vi "DashboardTest.vi"() -> ()   [LabVIEW 2020]
uses:
  <vilib>/Rock Robotics/Network Tables/NT Read Number.vi
  <vilib>/Rock Robotics/Network Tables/NT Read String.vi
  <vilib>/Rock Robotics/Network Tables/NT Read Boolean.vi
  <vilib>/vision/NI_Vision_Development_Module.lvlib
panel:
  out "Image 2":T1(plugin-control)
  out "Image":T1(plugin-control)
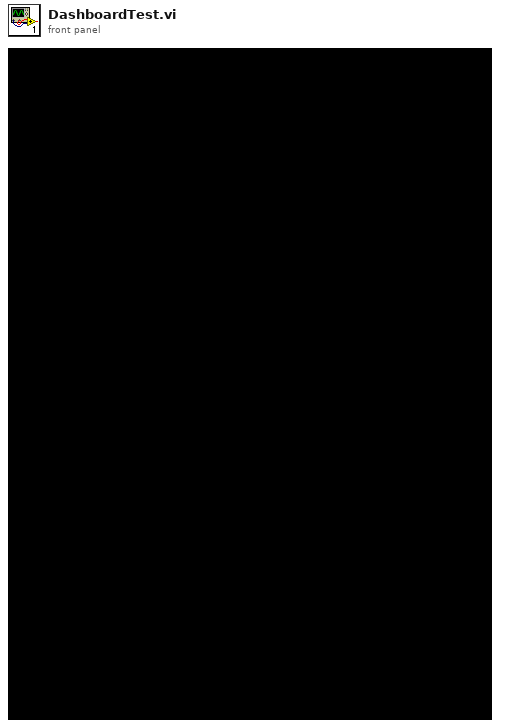
[diagram p1: front panel]
types:
  T1 = typedef "IMAQ Image.ctl" = refnum<image>
  T2 = typedef "Image Type" = u32
  T3 = typedef "LVRectTypeDef.ctl" = cluster{"Left":i16, "Top":i16, "Right":i16, "Bottom":i16}
  T4 = typedef "LVAllMonitorsDisplayTypeDef.ctl" = cluster{"Bounds":cluster{"Left":i16, "Top":i16, "Right":i16, "Bottom":i16}, "Depth":i16}[]
  T5 = cluster{"Left":i16, "Top":i16, "Right":i16, "Bottom":i16}
  T6 = cluster{"Bounds[0]":i16, "Bounds[1]":i16, "Bounds[2]":i16, "Bounds[3]":i16}
  T7 = cluster{"Left":i32, "Top":i32, "Right":i32, "Bottom":i32}
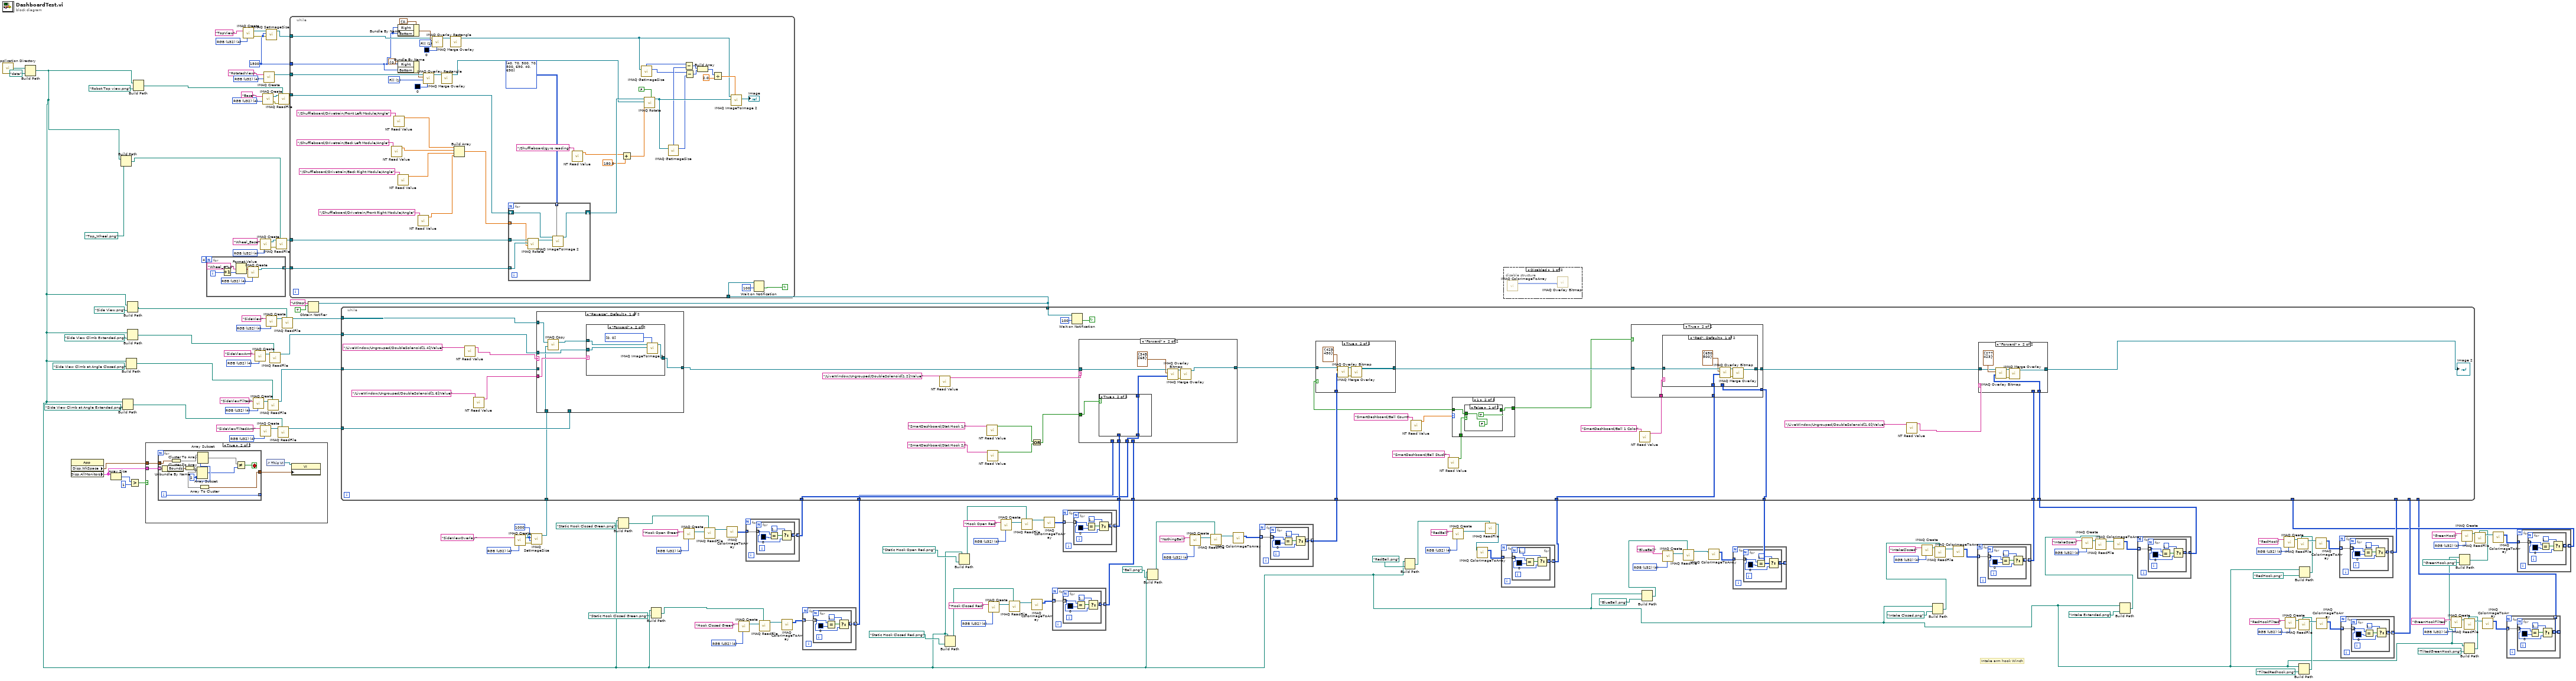
[diagram p0: block diagram]
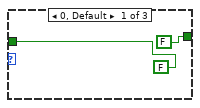
[diagram p4: hidden frame]
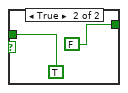
[diagram p5: hidden frame]
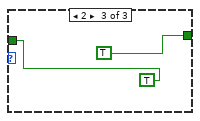
[diagram p6: hidden frame]
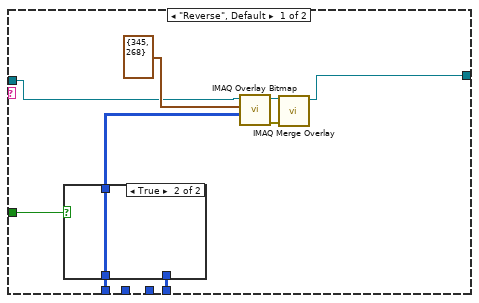
[diagram p7: hidden frame]
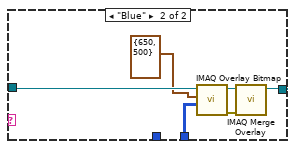
[diagram p11: hidden frame]
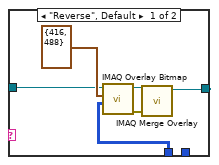
[diagram p12: hidden frame]
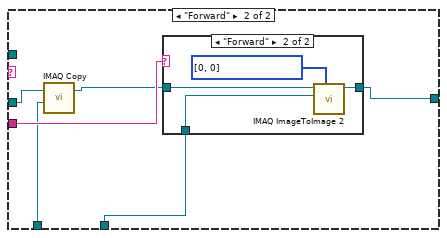
[diagram p15: hidden frame]
diagram:
  w11 = T2 4 items=["Grayscale (U8)", "Grayscale (I16)", "Grayscale (SGL)", "Complex (CSG)", "RGB (U32)", "HSL (U32)", "RGB (U64)", "Grayscale (U16)"] ("Image Type")
  w16 = T2 4 items=["Grayscale (U8)", "Grayscale (I16)", "Grayscale (SGL)", "Complex (CSG)", "RGB (U32)", "HSL (U32)", "RGB (U64)", "Grayscale (U16)"] ("Image Type")
  w32 = T2 4 items=["Grayscale (U8)", "Grayscale (I16)", "Grayscale (SGL)", "Complex (CSG)", "RGB (U32)", "HSL (U32)", "RGB (U64)", "Grayscale (U16)"] ("Image Type")
  w37 = T2 4 items=["Grayscale (U8)", "Grayscale (I16)", "Grayscale (SGL)", "Complex (CSG)", "RGB (U32)", "HSL (U32)", "RGB (U64)", "Grayscale (U16)"] ("Image Type")
  w42 = T2 4 items=["Grayscale (U8)", "Grayscale (I16)", "Grayscale (SGL)", "Complex (CSG)", "RGB (U32)", "HSL (U32)", "RGB (U64)", "Grayscale (U16)"] ("Image Type")
  w48 = T2 4 items=["Grayscale (U8)", "Grayscale (I16)", "Grayscale (SGL)", "Complex (CSG)", "RGB (U32)", "HSL (U32)", "RGB (U64)", "Grayscale (U16)"] ("Image Type")
  w64 = T2 4 items=["Grayscale (U8)", "Grayscale (I16)", "Grayscale (SGL)", "Complex (CSG)", "RGB (U32)", "HSL (U32)", "RGB (U64)", "Grayscale (U16)"] ("Image Type")
  w72 = T2 4 items=["Grayscale (U8)", "Grayscale (I16)", "Grayscale (SGL)", "Complex (CSG)", "RGB (U32)", "HSL (U32)", "RGB (U64)", "Grayscale (U16)"] ("Image Type")
  w102 = T2 4 items=["Grayscale (U8)", "Grayscale (I16)", "Grayscale (SGL)", "Complex (CSG)", "RGB (U32)", "HSL (U32)", "RGB (U64)", "Grayscale (U16)"] ("Image Type")
  w118 = T2 4 items=["Grayscale (U8)", "Grayscale (I16)", "Grayscale (SGL)", "Complex (CSG)", "RGB (U32)", "HSL (U32)", "RGB (U64)", "Grayscale (U16)"] ("Image Type")
  w121 = T2 4 items=["Grayscale (U8)", "Grayscale (I16)", "Grayscale (SGL)", "Complex (CSG)", "RGB (U32)", "HSL (U32)", "RGB (U64)", "Grayscale (U16)"] ("Image Type")
  w124 = T2 4 items=["Grayscale (U8)", "Grayscale (I16)", "Grayscale (SGL)", "Complex (CSG)", "RGB (U32)", "HSL (U32)", "RGB (U64)", "Grayscale (U16)"] ("Image Type")
  w127 = T2 4 items=["Grayscale (U8)", "Grayscale (I16)", "Grayscale (SGL)", "Complex (CSG)", "RGB (U32)", "HSL (U32)", "RGB (U64)", "Grayscale (U16)"] ("Image Type")
  w104 = 1000 ("Y Resolution")
  w133 = T2 4 items=["Grayscale (U8)", "Grayscale (I16)", "Grayscale (SGL)", "Complex (CSG)", "RGB (U32)", "HSL (U32)", "RGB (U64)", "Grayscale (U16)"] ("Image Type")
  w139 = T2 4 items=["Grayscale (U8)", "Grayscale (I16)", "Grayscale (SGL)", "Complex (CSG)", "RGB (U32)", "HSL (U32)", "RGB (U64)", "Grayscale (U16)"] ("Image Type")
  w142 = T2 4 items=["Grayscale (U8)", "Grayscale (I16)", "Grayscale (SGL)", "Complex (CSG)", "RGB (U32)", "HSL (U32)", "RGB (U64)", "Grayscale (U16)"] ("Image Type")
  w146 = T2 4 items=["Grayscale (U8)", "Grayscale (I16)", "Grayscale (SGL)", "Complex (CSG)", "RGB (U32)", "HSL (U32)", "RGB (U64)", "Grayscale (U16)"] ("Image Type")
  w148 = T2 4 items=["Grayscale (U8)", "Grayscale (I16)", "Grayscale (SGL)", "Complex (CSG)", "RGB (U32)", "HSL (U32)", "RGB (U64)", "Grayscale (U16)"] ("Image Type")
  w152 = T2 4 items=["Grayscale (U8)", "Grayscale (I16)", "Grayscale (SGL)", "Complex (CSG)", "RGB (U32)", "HSL (U32)", "RGB (U64)", "Grayscale (U16)"] ("Image Type")
  w163 = T2 4 items=["Grayscale (U8)", "Grayscale (I16)", "Grayscale (SGL)", "Complex (CSG)", "RGB (U32)", "HSL (U32)", "RGB (U64)", "Grayscale (U16)"] ("Image Type")
  w164 = T2 4 items=["Grayscale (U8)", "Grayscale (I16)", "Grayscale (SGL)", "Complex (CSG)", "RGB (U32)", "HSL (U32)", "RGB (U64)", "Grayscale (U16)"] ("Image Type")
  w150 = 1500 ("Y Resolution")
  w169 = T2 4 items=["Grayscale (U8)", "Grayscale (I16)", "Grayscale (SGL)", "Complex (CSG)", "RGB (U32)", "HSL (U32)", "RGB (U64)", "Grayscale (U16)"] ("Image Type")
  # "Intake arm hook Winch"
  n1 = call <vilib>:"Application Directory.vi"() -> ("Application Directory"=w97:path)
  n2 = Build Path(base path=w97, name or relative path=path "data") -> (appended path=w5:path)
  n3 = property class="App"() -> ("Disp.WkSpace"=w53:T3, "Disp.AllMonitors"=w54:T4)  [unwired: 2 in, 2 out]
  n4 = Array Size(array=w54) -> (size(s)=w57:i32)
  n5 = Build Path(base path=w5, name or relative path=path "Top_Wheel.png") -> (appended path=w92:path)
  n6 = Build Path(base path=w5, name or relative path=path "Side View Climb at Angle Extended.png") -> (appended path=w84:path)
  n7 = Build Path(base path=w5, name or relative path=path "Side View Climb at Angle Closed.png") -> (appended path=w86:path)
  n8 = Build Path(base path=w5, name or relative path=path "Side View.png") -> (appended path=w90:path)
  n9 = Build Path(base path=w5, name or relative path=path "Side View Climb Extended.png") -> (appended path=w88:path)
  n10 = Greater?(x=w57, y=1) -> (0:w55:bool)
  n11 = Build Path(base path=w5, name or relative path=path "Robot Top view.png") -> (appended path=w94:path)
  n12 = case shown="True" w55 {
    tunnel: w54 -> [_ w174]
    tunnel: w53 -> [_ w173]
    frame False {
    }
    frame True {
      n13 = for {
        tunnel: w174 -> [w182] mode=indexing
        tunnel: w173 -> [w183]
        tunnel: [w175] -> w171
        tunnel: [w184] -> _ mode=indexing
        i -> [w184]
        stop <- w185 stop-if-true
        w179 = 2 ("length")
        n14 = Unbundle By Name(w182) -> ("Bounds"=w181:T5)
        n15 = Cluster To Array(cluster=w183) -> (array=w180:i16[])
        n16 = Cluster To Array(cluster=w181) -> (array=w176:i16[])
        n17 = Array Subset(array=w176, length=w179) -> (w177:i16[])  [unwired: 1 in]
        n18 = Array Subset(array=w180, length=w179) -> (w178:i16[])  [unwired: 1 in]
        n19 = Array To Cluster(array=w176) -> (cluster=w175:T6)
        n20 = Not Equal?(x=w178, y=w177) -> (x != y?=w185:bool)
      }
      n21 = control-ref of="This VI"() -> (w172:refnum<vi>)
      n22 = property class="VI"(reference=w172, "Front Panel.WinBounds"=w171) -> ()  [unwired: 1 in, 2 out]
    }
  }
  n23 = for {
    N: 4 -> [_]
    tunnel: [w186] -> w154 mode=indexing
    i -> [w188]
    w191 = T2 4 items=["Grayscale (U8)", "Grayscale (I16)", "Grayscale (SGL)", "Complex (CSG)", "RGB (U32)", "HSL (U32)", "RGB (U64)", "Grayscale (U16)"] ("Image Type")
    n24 = Increment(x=w188) -> (x+1=w187:i32)
    n25 = Format Value(format string="Wheel_#%d" ("Image Name"), value (0)=w187) -> (output string=w190:string)  [unwired: 1 in]
    n26 = call "IMAQ Create"("Image Name"=w190, "Image Type"=w191) -> ("New Image"=w186:T1)  [unwired: 3 in, 1 out]
  }
  n27 = call "IMAQ Create"("Image Name"="TopView", "Image Type"=w169) -> ("New Image"=w168:T1, "error out"=w167:errorcluster)  [unwired: 3 in]
  n28 = call "IMAQ Create"("Image Name"="SideViewTilted", "Image Type"=w146) -> ("New Image"=w145:T1)  [unwired: 3 in, 1 out]
  n29 = call "IMAQ Create"("Image Name"="SideViewArm", "Image Type"=w142) -> ("New Image"=w141:T1)  [unwired: 3 in, 1 out]
  n30 = call "IMAQ Create"("Image Name"="Wheel_Base", "Image Type"=w164) -> ("New Image"=w160:T1, "error out"=w161:errorcluster)  [unwired: 3 in]
  n31 = call "IMAQ Create"("Image Name"="SideViewTiltedArm", "Image Type"=w139) -> ("New Image"=w138:T1)  [unwired: 3 in, 1 out]
  n32 = call "IMAQ Create"("Image Name"="Base", "Image Type"=w163) -> ("New Image"=w158:T1, "error out"=w159:errorcluster)  [unwired: 3 in]
  n33 = call "IMAQ Create"("Image Name"="RotatedView", "Image Type"=w152) -> ("New Image"=w151:T1)  [unwired: 3 in, 1 out]
  n34 = call "IMAQ SetImageSize"("error in (no error)"=w167, "Y Resolution"=w150, "X Resolution"=w150, "Image"=w168) -> ("Image Out"=w166:T1)  [unwired: 1 in, 1 out]
  n35 = call "IMAQ Create"("Image Name"="SideView", "Image Type"=w148) -> ("New Image"=w144:T1)  [unwired: 3 in, 1 out]
  n36 = call "IMAQ ReadFile"("File Path"=w86, "Image"=w145) -> ("Image Out"=w137:T1)  [unwired: 5 in, 4 out]
  n37 = call "IMAQ ReadFile"("File Path"=w88, "Image"=w141) -> ("Image Out"=w136:T1)  [unwired: 5 in, 4 out]
  n38 = call "IMAQ ReadFile"("File Path"=w92, "error in (no error)"=w161, "Image"=w160) -> ("Image Out"=w156:T1)  [unwired: 4 in, 4 out]
  n39 = call "IMAQ ReadFile"("File Path"=w84, "Image"=w138) -> ("Image Out"=w135:T1)  [unwired: 5 in, 4 out]
  n40 = call "IMAQ ReadFile"("File Path"=w94, "error in (no error)"=w159, "Image"=w158) -> ("Image Out"=w157:T1)  [unwired: 4 in, 4 out]
  n41 = call "IMAQ ReadFile"("File Path"=w90, "Image"=w144) -> ("Image Out"=w129:T1)  [unwired: 5 in, 4 out]
  n42 = Obtain Notifier(name (unnamed)="UIStop", notification data type=TRUE) -> (notifier out=w50:refnum<notifier>)  [unwired: 2 in, 2 out]
  n43 = while {
    tunnel: w166 -> [w209]
    tunnel: w157 -> [w236]
    tunnel: w156 -> [w239]
    tunnel: w154 -> [w237]
    tunnel: w151 -> [w231]
    tunnel: w150 -> [w207]
    tunnel: w50 -> [w194]
    stop <- w192 continue-if-true
    w211 = u32 1 items=["Frame", "Fill", "Highlight"] ("Drawing Mode (Frame)")
    w219 = u32 1 items=["Frame", "Fill", "Highlight"] ("Drawing Mode (Frame)")
    n44 = call-poly <vilib>:"NT Read Value.vi"("Name"="/Shuffleboard/Drivetrain/Back Left Module/Angle") -> ("Numeric"=w201:dbl)  [unwired: 9 in, 1 out]
    n45 = call-poly <vilib>:"NT Read Value.vi"("Name"="/Shuffleboard/Drivetrain/Front Left Module/Angle") -> ("Numeric"=w197:dbl)  [unwired: 9 in, 1 out]
    n46 = Bundle By Name(cluster=T7 {"Left"=0, "Top"=0, "Right"=0, "Bottom"=0} ("Rectangle"), "Right"=w207, "Bottom"=w207) -> (w213:T7)
    n47 = Bundle By Name(cluster=T7 {"Left"=0, "Top"=0, "Right"=0, "Bottom"=0} ("Rectangle"), "Right"=w207, "Bottom"=w207) -> (w217:T7)
    n48 = call-poly <vilib>:"NT Read Value.vi"("Name"="/Shuffleboard/Drivetrain/Back Right Module/Angle") -> ("Numeric"=w199:dbl)  [unwired: 9 in, 1 out]
    n49 = call-poly <vilib>:"NT Read Value.vi"("Name"="/Shuffleboard/Drivetrain/Front Right Module/Angle") -> ("Numeric"=w203:dbl)  [unwired: 9 in, 1 out]
    n50 = call "IMAQ Overlay Rectangle"("Color"=u32 0, "Drawing Mode (Frame)"=w219, "Rectangle"=w217, "Image"=w231) -> ("Image Out"=w215:T1)  [unwired: 6 in, 1 out]
    n51 = call "IMAQ Overlay Rectangle"("Color"=u32 0, "Drawing Mode (Frame)"=w211, "Rectangle"=w213, "Image"=w209) -> ("Image Out"=w214:T1)  [unwired: 6 in, 1 out]
    n52 = call "IMAQ Merge Overlay"("Image Src"=w215) -> ("Image Dst Out"=w216:T1)  [unwired: 9 in, 1 out]
    n53 = call "IMAQ Merge Overlay"("Image Src"=w214) -> ("Image Dst Out"=w208:T1)  [unwired: 9 in, 1 out]
    n54 = Build Array(w197, w201, w199, w203) -> (w238:dbl[])
    n55 = for {
      tunnel: w238 -> [w244] mode=indexing
      tunnel: w237 -> [w245] mode=indexing
      tunnel: w239 -> [w246]
      shift-right: [w240] -> w234
      shift-left: w236 -> [w243]
      tunnel: i32[][] [[40, 70], [500, 70], [500, 690], [40, 690]] ("Offset Left/Top") -> [w241] mode=indexing
      n56 = call "IMAQ Rotate"("Angle (degrees)"=w244, "Image Dst"=w245, "Image Src"=w246) -> ("Image Dst Out"=w242:T1)  [unwired: 7 in, 1 out]
      n57 = call "IMAQ ImageToImage 2"("Offset Left/Top"=w241, "Image Src (Small)"=w242, "Image Src (Large)"=w243) -> ("Image Dst Out"=w240:T1)  [unwired: 7 in, 1 out]
    }
    n58 = call-poly <vilib>:"NT Read Value.vi"("Name"="/Shuffleboard/gyro reading") -> ("Numeric"=w195:dbl)  [unwired: 9 in, 1 out]
    n59 = Add(x=w195, y=180.0) -> (x+y=w206:dbl)
    n60 = call "IMAQ GetImageSize"("Image"=w208) -> ("Y Resolution"=w225:i32, "X Resolution"=w228:i32)  [unwired: 3 in, 1 out]
    n61 = call "IMAQ Rotate"("Maintain Size"=FALSE, "Angle (degrees)"=w206, "Image Dst"=w216, "Image Src"=w234) -> ("Image Dst Out"=w230:T1)  [unwired: 6 in, 1 out]
    n62 = call "IMAQ GetImageSize"("Image"=w230) -> ("Y Resolution"=w226:i32, "X Resolution"=w229:i32)  [unwired: 3 in, 1 out]
    n63 = Subtract(x=w228, y=w229) -> (x-y=w223:i32)
    n64 = Subtract(x=w225, y=w226) -> (x-y=w224:i32)
    n65 = Build Array(w223, w224) -> (w222:i32[])
    n66 = Divide(x=w222, y=2.0) -> (x/y=w221:dbl[])
    n67 = call "IMAQ ImageToImage 2"("Offset Left/Top"=w221, "Image Src (Small)"=w230, "Image Src (Large)"=w208) -> ("Image Dst Out"=→"Image":T1)  [unwired: 7 in, 1 out]
    n68 = Wait on Notification(notifier=w194, timeout in ms (-1)=100) -> (timed out?=w192:bool)  [unwired: 2 in, 3 out]
  }
  n69 = call "IMAQ Create"("Image Name"="SideViewOverlay", "Image Type"=w133) -> ("New Image"=w132:T1, "error out"=w131:errorcluster)  [unwired: 3 in]
  n70 = call "IMAQ SetImageSize"("error in (no error)"=w131, "Y Resolution"=w104, "X Resolution"=w104, "Image"=w132) -> ("Image Out"=w130:T1)  [unwired: 1 in, 1 out]
  n71 = Build Path(base path=w5, name or relative path=path "Static Hook Closed Green.png") -> (appended path=w6:path)
  n72 = Build Path(base path=w5, name or relative path=path "Static Hook Closed Green.png") -> (appended path=w7:path)
  n73 = call "IMAQ Create"("Image Name"="Hook Open Green", "Image Type"=w11) -> ("New Image"=w10:T1)  [unwired: 3 in, 1 out]
  n74 = call "IMAQ ReadFile"("File Path"=w6, "Image"=w10) -> ("Image Out"=w9:T1)  [unwired: 5 in, 4 out]
  n75 = call "IMAQ ColorImageToArray"("Image"=w9) -> ("Image Pixels (U32)"=w8:u32[][])  [unwired: 3 in, 2 out]
  n76 = call "IMAQ Create"("Image Name"="Hook Closed Green", "Image Type"=w16) -> ("New Image"=w15:T1)  [unwired: 3 in, 1 out]
  n77 = for {
    tunnel: w8 -> [w248] mode=indexing
    tunnel: [w247] -> w2 mode=indexing
    n78 = for {
      tunnel: w248 -> [w251] mode=indexing
      tunnel: [w249] -> w247 mode=indexing
      n79 = Equal?(x=w251, y=u32 0) -> (x = y?=w252:bool)
      n80 = Select(t=u32 16777216, s=w252, f=w251) -> (s? t:f=w249:u32)
    }
  }
  n81 = call "IMAQ ReadFile"("File Path"=w7, "Image"=w15) -> ("Image Out"=w14:T1)  [unwired: 5 in, 4 out]
  n82 = call "IMAQ ColorImageToArray"("Image"=w14) -> ("Image Pixels (U32)"=w13:u32[][])  [unwired: 3 in, 2 out]
  n83 = for {
    tunnel: w13 -> [w255] mode=indexing
    tunnel: [w254] -> w1 mode=indexing
    n84 = for {
      tunnel: w255 -> [w258] mode=indexing
      tunnel: [w256] -> w254 mode=indexing
      n85 = Equal?(x=w258, y=u32 0) -> (x = y?=w259:bool)
      n86 = Select(t=u32 16777216, s=w259, f=w258) -> (s? t:f=w256:u32)
    }
  }
  n87 = Build Path(base path=w5, name or relative path=path "Static Hook Closed Red.png") -> (appended path=w60:path)
  n88 = Build Path(base path=w5, name or relative path=path "Static Hook Open Red.png") -> (appended path=w68:path)
  n89 = call "IMAQ Create"("Image Name"="Hook Closed Red", "Image Type"=w64) -> ("New Image"=w63:T1)  [unwired: 3 in, 1 out]
  n90 = call "IMAQ Create"("Image Name"="Hook Open Red", "Image Type"=w72) -> ("New Image"=w71:T1)  [unwired: 3 in, 1 out]
  n91 = call "IMAQ ReadFile"("File Path"=w60, "Image"=w63) -> ("Image Out"=w62:T1)  [unwired: 5 in, 4 out]
  n92 = call "IMAQ ReadFile"("File Path"=w68, "Image"=w71) -> ("Image Out"=w70:T1)  [unwired: 5 in, 4 out]
  n93 = call "IMAQ ColorImageToArray"("Image"=w62) -> ("Image Pixels (U32)"=w61:u32[][])  [unwired: 3 in, 2 out]
  n94 = call "IMAQ ColorImageToArray"("Image"=w70) -> ("Image Pixels (U32)"=w69:u32[][])  [unwired: 3 in, 2 out]
  n95 = for {
    tunnel: w61 -> [w262] mode=indexing
    tunnel: [w261] -> w58 mode=indexing
    n96 = for {
      tunnel: w262 -> [w265] mode=indexing
      tunnel: [w263] -> w261 mode=indexing
      n97 = Equal?(x=w265, y=u32 0) -> (x = y?=w266:bool)
      n98 = Select(t=u32 16777216, s=w266, f=w265) -> (s? t:f=w263:u32)
    }
  }
  n99 = for {
    tunnel: w69 -> [w269] mode=indexing
    tunnel: [w268] -> w66 mode=indexing
    n100 = for {
      tunnel: w269 -> [w272] mode=indexing
      tunnel: [w270] -> w268 mode=indexing
      n101 = Equal?(x=w272, y=u32 0) -> (x = y?=w273:bool)
      n102 = Select(t=u32 16777216, s=w273, f=w272) -> (s? t:f=w270:u32)
    }
  }
  n103 = Build Path(base path=w5, name or relative path=path "Ball.png") -> (appended path=w82:path)
  n104 = call "IMAQ Create"("Image Name"="NothingBall", "Image Type"=w124) -> ("New Image"=w123:T1)  [unwired: 3 in, 1 out]
  n105 = call "IMAQ ReadFile"("File Path"=w82, "Image"=w123) -> ("Image Out"=w116:T1)  [unwired: 5 in, 4 out]
  n106 = call "IMAQ ColorImageToArray"("Image"=w116) -> ("Image Pixels (U32)"=w115:u32[][])  [unwired: 3 in, 2 out]
  n107 = for {
    tunnel: w115 -> [w276] mode=indexing
    tunnel: [w275] -> w108 mode=indexing
    n108 = for {
      tunnel: w276 -> [w279] mode=indexing
      tunnel: [w277] -> w275 mode=indexing
      n109 = Equal?(x=w279, y=u32 0) -> (x = y?=w280:bool)
      n110 = Select(t=u32 16777216, s=w280, f=w279) -> (s? t:f=w277:u32)
    }
  }
  n111 = Build Path(base path=w5, name or relative path=path "RedBall.png") -> (appended path=w80:path)
  n112 = call "IMAQ Create"("Image Name"="RedBall", "Image Type"=w121) -> ("New Image"=w120:T1)  [unwired: 3 in, 1 out]
  n113 = call "IMAQ ReadFile"("File Path"=w80, "Image"=w120) -> ("Image Out"=w113:T1)  [unwired: 5 in, 4 out]
  n114 = call "IMAQ ColorImageToArray"("Image"=w113) -> ("Image Pixels (U32)"=w114:u32[][])  [unwired: 3 in, 2 out]
  n115 = for {
    tunnel: w114 -> [w283] mode=indexing
    tunnel: [w282] -> w109 mode=indexing
    n116 = for {
      tunnel: w283 -> [w286] mode=indexing
      tunnel: [w284] -> w282 mode=indexing
      n117 = Equal?(x=w286, y=u32 0) -> (x = y?=w287:bool)
      n118 = Select(t=u32 16777216, s=w287, f=w286) -> (s? t:f=w284:u32)
    }
  }
  n119 = disable-structure shown="Disabled" {
    frame Disabled {
      n120 = call "IMAQ ColorImageToArray"() -> ("Image Pixels (U32)"=w289:u32[][])  [unwired: 4 in, 2 out]
      n121 = call "IMAQ Overlay Bitmap"("Bitmap"=w289) -> ()  [unwired: 9 in, 2 out]
    }
    frame Enabled {
    }
  }
  n122 = Build Path(base path=w5, name or relative path=path "BlueBall.png") -> (appended path=w79:path)
  n123 = call "IMAQ Create"("Image Name"="BlueBall", "Image Type"=w118) -> ("New Image"=w117:T1)  [unwired: 3 in, 1 out]
  n124 = call "IMAQ ReadFile"("File Path"=w79, "Image"=w117) -> ("Image Out"=w111:T1)  [unwired: 5 in, 4 out]
  n125 = call "IMAQ ColorImageToArray"("Image"=w111) -> ("Image Pixels (U32)"=w112:u32[][])  [unwired: 3 in, 2 out]
  n126 = for {
    tunnel: w112 -> [w291] mode=indexing
    tunnel: [w290] -> w110 mode=indexing
    n127 = for {
      tunnel: w291 -> [w294] mode=indexing
      tunnel: [w292] -> w290 mode=indexing
      n128 = Equal?(x=w294, y=u32 0) -> (x = y?=w295:bool)
      n129 = Select(t=u32 16777216, s=w295, f=w294) -> (s? t:f=w292:u32)
    }
  }
  n130 = call "IMAQ Create"("Image Name"="IntakeClosed", "Image Type"=w127) -> ("New Image"=w126:T1)  [unwired: 3 in, 1 out]
  n131 = Build Path(base path=w5, name or relative path=path "Intake Closed.png") -> (appended path=w78:path)
  n132 = call "IMAQ ReadFile"("File Path"=w78, "Image"=w126) -> ("Image Out"=w106:T1)  [unwired: 5 in, 4 out]
  n133 = call "IMAQ ColorImageToArray"("Image"=w106) -> ("Image Pixels (U32)"=w107:u32[][])  [unwired: 3 in, 2 out]
  n134 = for {
    tunnel: w107 -> [w298] mode=indexing
    tunnel: [w297] -> w105 mode=indexing
    n135 = for {
      tunnel: w298 -> [w301] mode=indexing
      tunnel: [w299] -> w297 mode=indexing
      n136 = Equal?(x=w301, y=u32 0) -> (x = y?=w302:bool)
      n137 = Select(t=u32 16777216, s=w302, f=w301) -> (s? t:f=w299:u32)
    }
  }
  n138 = call "IMAQ Create"("Image Name"="IntakeOpen", "Image Type"=w102) -> ("New Image"=w101:T1)  [unwired: 3 in, 1 out]
  n139 = Build Path(base path=w5, name or relative path=path "Intake Extended.png") -> (appended path=w77:path)
  n140 = call "IMAQ ReadFile"("File Path"=w77, "Image"=w101) -> ("Image Out"=w99:T1)  [unwired: 5 in, 4 out]
  n141 = call "IMAQ ColorImageToArray"("Image"=w99) -> ("Image Pixels (U32)"=w100:u32[][])  [unwired: 3 in, 2 out]
  n142 = for {
    tunnel: w100 -> [w305] mode=indexing
    tunnel: [w304] -> w98 mode=indexing
    n143 = for {
      tunnel: w305 -> [w308] mode=indexing
      tunnel: [w306] -> w304 mode=indexing
      n144 = Equal?(x=w308, y=u32 0) -> (x = y?=w309:bool)
      n145 = Select(t=u32 16777216, s=w309, f=w308) -> (s? t:f=w306:u32)
    }
  }
  n146 = call "IMAQ Create"("Image Name"="RedHook", "Image Type"=w48) -> ("New Image"=w47:T1)  [unwired: 3 in, 1 out]
  n147 = call "IMAQ Create"("Image Name"="RedHookTilted", "Image Type"=w42) -> ("New Image"=w41:T1)  [unwired: 3 in, 1 out]
  n148 = Build Path(base path=w5, name or relative path=path "TiltedRedhook.png") -> (appended path=w25:path)
  n149 = call "IMAQ ReadFile"("File Path"=w25, "Image"=w41) -> ("Image Out"=w39:T1)  [unwired: 5 in, 4 out]
  n150 = Build Path(base path=w5, name or relative path=path "RedHook.png") -> (appended path=w24:path)
  n151 = call "IMAQ ReadFile"("File Path"=w24, "Image"=w47) -> ("Image Out"=w45:T1)  [unwired: 5 in, 4 out]
  n152 = call "IMAQ ColorImageToArray"("Image"=w45) -> ("Image Pixels (U32)"=w46:u32[][])  [unwired: 3 in, 2 out]
  n153 = call "IMAQ ColorImageToArray"("Image"=w39) -> ("Image Pixels (U32)"=w40:u32[][])  [unwired: 3 in, 2 out]
  n154 = for {
    tunnel: w46 -> [w312] mode=indexing
    tunnel: [w311] -> w44 mode=indexing
    n155 = for {
      tunnel: w312 -> [w315] mode=indexing
      tunnel: [w313] -> w311 mode=indexing
      n156 = Equal?(x=w315, y=u32 0) -> (x = y?=w316:bool)
      n157 = Select(t=u32 16777216, s=w316, f=w315) -> (s? t:f=w313:u32)
    }
  }
  n158 = for {
    tunnel: w40 -> [w319] mode=indexing
    tunnel: [w318] -> w28 mode=indexing
    n159 = for {
      tunnel: w319 -> [w322] mode=indexing
      tunnel: [w320] -> w318 mode=indexing
      n160 = Equal?(x=w322, y=u32 0) -> (x = y?=w323:bool)
      n161 = Select(t=u32 16777216, s=w323, f=w322) -> (s? t:f=w320:u32)
    }
  }
  n162 = call "IMAQ Create"("Image Name"="GreenHookTilted", "Image Type"=w32) -> ("New Image"=w31:T1)  [unwired: 3 in, 1 out]
  n163 = Build Path(base path=w5, name or relative path=path "GreenHook.png") -> (appended path=w22:path)
  n164 = call "IMAQ Create"("Image Name"="GreenHook", "Image Type"=w37) -> ("New Image"=w36:T1)  [unwired: 3 in, 1 out]
  n165 = Build Path(base path=w5, name or relative path=path "TiltedGreenHook.png") -> (appended path=w23:path)
  n166 = call "IMAQ ReadFile"("File Path"=w23, "Image"=w31) -> ("Image Out"=w29:T1)  [unwired: 5 in, 4 out]
  n167 = call "IMAQ ReadFile"("File Path"=w22, "Image"=w36) -> ("Image Out"=w34:T1)  [unwired: 5 in, 4 out]
  n168 = call "IMAQ ColorImageToArray"("Image"=w29) -> ("Image Pixels (U32)"=w30:u32[][])  [unwired: 3 in, 2 out]
  n169 = call "IMAQ ColorImageToArray"("Image"=w34) -> ("Image Pixels (U32)"=w35:u32[][])  [unwired: 3 in, 2 out]
  n170 = for {
    tunnel: w30 -> [w326] mode=indexing
    tunnel: [w325] -> _ mode=indexing
    tunnel: [w325] -> w26 mode=indexing
    n171 = for {
      tunnel: w326 -> [w329] mode=indexing
      tunnel: [w327] -> w325 mode=indexing
      n172 = Equal?(x=w329, y=u32 0) -> (x = y?=w330:bool)
      n173 = Select(t=u32 16777216, s=w330, f=w329) -> (s? t:f=w327:u32)
    }
  }
  n174 = for {
    tunnel: w35 -> [w333] mode=indexing
    tunnel: [w332] -> w27 mode=indexing
    n175 = for {
      tunnel: w333 -> [w336] mode=indexing
      tunnel: [w334] -> w332 mode=indexing
      n176 = Equal?(x=w336, y=u32 0) -> (x = y?=w337:bool)
      n177 = Select(t=u32 16777216, s=w337, f=w336) -> (s? t:f=w334:u32)
    }
  }
  n178 = while {
    tunnel: w129 -> [w379]
    tunnel: w137 -> [w377]
    tunnel: w136 -> [w381]
    tunnel: w135 -> [w380]
    tunnel: w130 -> [w378]
    tunnel: w110 -> [w375]
    tunnel: w109 -> [w374]
    tunnel: w108 -> [w373]
    tunnel: w105 -> [w372]
    tunnel: w98 -> [w370]
    tunnel: w66 -> [w369]
    tunnel: w58 -> [w346]
    tunnel: w50 -> [w354]
    tunnel: w44 -> [_]
    tunnel: w28 -> [_]
    tunnel: w27 -> [_]
    tunnel: w26 -> [_]
    tunnel: w2 -> [w348]
    tunnel: w1 -> [w347]
    stop <- w353 continue-if-true
    n179 = call-poly <vilib>:"NT Read Value.vi"("Name"="/LiveWindow/Ungrouped/DoubleSolenoid[1,4]/Value") -> ("String"=w344:string)  [unwired: 9 in, 1 out]
    n180 = call-poly <vilib>:"NT Read Value.vi"("Name"="/LiveWindow/Ungrouped/DoubleSolenoid[1,6]/Value") -> ("String"=w350:string)  [unwired: 9 in, 1 out]
    n181 = case shown="\"Reverse\", Default" w344 {
      tunnel: w350 -> [w457 w468]
      tunnel: [w452 w467] -> w345
      tunnel: w381 -> [w456 _]
      tunnel: w380 -> [_ w466]
      tunnel: w379 -> [w455 _]
      tunnel: w378 -> [w454 w465]
      tunnel: w377 -> [_ w464]
      frame "Reverse", Default {
        n182 = call "IMAQ Copy"("Image Dst"=w454, "Image Src"=w455) -> ("Image Dst Out"=w453:T1)  [unwired: 4 in, 1 out]
        n183 = case shown="\"Forward\"" w457 {
          tunnel: [w458 w459] -> w452
          tunnel: w453 -> [w458 w460]
          tunnel: w456 -> [_ w462]
          frame "Reverse", Default {
          }
          frame "Forward" {
            n184 = call "IMAQ ImageToImage 2"("Offset Left/Top"=i32[] [0, 0], "Image Src (Small)"=w462, "Image Src (Large)"=w460) -> ("Image Dst Out"=w459:T1)  [unwired: 7 in, 1 out]
          }
        }
      }
      frame "Forward" {
        n185 = call "IMAQ Copy"("Image Dst"=w465, "Image Src"=w464) -> ("Image Dst Out"=w463:T1)  [unwired: 4 in, 1 out]
        n186 = case shown="\"Forward\"" w468 {
          tunnel: [w469 w471] -> w467
          tunnel: w463 -> [w469 w470]
          tunnel: w466 -> [_ w472]
          frame "Reverse", Default {
          }
          frame "Forward" {
            n187 = call "IMAQ ImageToImage 2"("Offset Left/Top"=i32[] [0, 0], "Image Src (Small)"=w472, "Image Src (Large)"=w470) -> ("Image Dst Out"=w471:T1)  [unwired: 7 in, 1 out]
          }
        }
      }
    }
    n188 = call-poly <vilib>:"NT Read Value.vi"("Name"="/LiveWindow/Ungrouped/DoubleSolenoid[1,2]/Value") -> ("String"=w349:string)  [unwired: 9 in, 1 out]
    n189 = call-poly <vilib>:"NT Read Value.vi"("Name"="SmartDashboard/Stat Hook 1/") -> ("Boolean"=w341:bool)  [unwired: 9 in, 1 out]
    n190 = call-poly <vilib>:"NT Read Value.vi"("Name"="SmartDashboard/Stat Hook 2/") -> ("Boolean"=w340:bool)  [unwired: 9 in, 1 out]
    n191 = Or(x=w341, y=w340) -> (x .or. y?=w339:bool)
    n192 = Wait on Notification(notifier=w354, timeout in ms (-1)=100) -> (timed out?=w353:bool)  [unwired: 2 in, 3 out]
    n193 = case shown="\"Forward\"" w349 {
      tunnel: w369 -> [_ w408]
      tunnel: [w398 w409] -> w368
      tunnel: w348 -> [_ w406]
      tunnel: w347 -> [w397 _]
      tunnel: w346 -> [w395 _]
      tunnel: w345 -> [w394 w405]
      tunnel: w339 -> [w393 w404]
      frame "Reverse", Default {
        n194 = case shown="True" w393 {
          tunnel: w397 -> [_ w403]
          tunnel: [w402 w403] -> w396
          tunnel: w395 -> [w402 _]
          frame False {
          }
          frame True {
          }
        }
        n195 = call "IMAQ Overlay Bitmap"("Bitmap"=w396, "Top Left Point"=cluster{"X":i32, "Y":i32} {"X"=345, "Y"=268}, "Image"=w394) -> ("error out"=w401:errorcluster, "Image Out"=w400:T1)  [unwired: 7 in]
        n196 = call "IMAQ Merge Overlay"("error in (no error)"=w401, "Image Src"=w400) -> ("Image Dst Out"=w398:T1)  [unwired: 8 in, 1 out]
      }
      frame "Forward" {
        n197 = case shown="True" w404 {
          tunnel: [w413 w414] -> w407
          tunnel: w408 -> [w413 _]
          tunnel: w406 -> [_ w414]
          frame False {
          }
          frame True {
          }
        }
        n198 = call "IMAQ Overlay Bitmap"("Bitmap"=w407, "Top Left Point"=cluster{"X":i32, "Y":i32} {"X"=345, "Y"=268}, "Image"=w405) -> ("error out"=w412:errorcluster, "Image Out"=w411:T1)  [unwired: 7 in]
        n199 = call "IMAQ Merge Overlay"("error in (no error)"=w412, "Image Src"=w411) -> ("Image Dst Out"=w409:T1)  [unwired: 8 in, 1 out]
      }
    }
    n200 = call-poly <vilib>:"NT Read Value.vi"("Name"="SmartDashboard/Ball Count") -> ("Numeric"=w365:dbl)  [unwired: 9 in, 1 out]
    n201 = call-poly <vilib>:"NT Read Value.vi"("Name"="SmartDashboard/Ball Stuck") -> ("Boolean"=w363:bool)  [unwired: 9 in, 1 out]
    n202 = case shown="1" w365 {
      tunnel: [FALSE w386 TRUE] -> w361
      tunnel: [FALSE w385 TRUE] -> w362
      tunnel: w363 -> [_ w384 _]
      frame 0, Default {
      }
      frame 1 {
        n203 = case shown="False" w384 {
          tunnel: [FALSE TRUE] -> w386
          tunnel: [TRUE FALSE] -> w385
          frame False {
          }
          frame True {
          }
        }
      }
      frame 2 {
      }
    }
    n204 = case shown="True" w361 {
      tunnel: w368 -> [w445 w450]
      tunnel: [w445 w451] -> w371
      tunnel: w373 -> [_ w449]
      frame False {
      }
      frame True {
        n205 = call "IMAQ Overlay Bitmap"("Bitmap"=w449, "Top Left Point"=cluster{"X":i32, "Y":i32} {"X"=425, "Y"=450}, "Image"=w450) -> ("error out"=w448:errorcluster, "Image Out"=w447:T1)  [unwired: 7 in]
        n206 = call "IMAQ Merge Overlay"("error in (no error)"=w448, "Image Src"=w447) -> ("Image Dst Out"=w451:T1)  [unwired: 8 in, 1 out]
      }
    }
    n207 = call-poly <vilib>:"NT Read Value.vi"("Name"="SmartDashboard/Ball 1 Color") -> ("String"=w358:string)  [unwired: 9 in, 1 out]
    n208 = case shown="True" w362 {
      tunnel: w371 -> [w415 w420]
      tunnel: [w415 w419] -> w376
      tunnel: w375 -> [_ w418]
      tunnel: w374 -> [_ w417]
      tunnel: w358 -> [_ w416]
      frame False {
      }
      frame True {
        n209 = case shown="\"Red\", Default" w416 {
          tunnel: w420 -> [w426 w431]
          tunnel: [w425 w432] -> w419
          tunnel: w418 -> [_ w430]
          tunnel: w417 -> [w424 _]
          frame "Red", Default {
            n210 = call "IMAQ Overlay Bitmap"("Bitmap"=w424, "Top Left Point"=cluster{"X":i32, "Y":i32} {"X"=650, "Y"=500}, "Image"=w426) -> ("error out"=w422:errorcluster, "Image Out"=w421:T1)  [unwired: 7 in]
            n211 = call "IMAQ Merge Overlay"("error in (no error)"=w422, "Image Src"=w421) -> ("Image Dst Out"=w425:T1)  [unwired: 8 in, 1 out]
          }
          frame "Blue" {
            n212 = call "IMAQ Overlay Bitmap"("Bitmap"=w430, "Top Left Point"=cluster{"X":i32, "Y":i32} {"X"=650, "Y"=500}, "Image"=w431) -> ("error out"=w429:errorcluster, "Image Out"=w428:T1)  [unwired: 7 in]
            n213 = call "IMAQ Merge Overlay"("error in (no error)"=w429, "Image Src"=w428) -> ("Image Dst Out"=w432:T1)  [unwired: 8 in, 1 out]
          }
        }
      }
    }
    n214 = call-poly <vilib>:"NT Read Value.vi"("Name"="/LiveWindow/Ungrouped/DoubleSolenoid[1,0]/Value") -> ("String"=w357:string)  [unwired: 9 in, 1 out]
    n215 = case shown="\"Forward\"" w357 {
      tunnel: w376 -> [w434 w441]
      tunnel: [w433 w440] -> w351
      tunnel: w372 -> [w436 _]
      tunnel: w370 -> [_ w439]
      frame "Reverse", Default {
        n216 = call "IMAQ Overlay Bitmap"("Bitmap"=w436, "Top Left Point"=cluster{"X":i32, "Y":i32} {"X"=416, "Y"=488}, "Image"=w434) -> ("error out"=w438:errorcluster, "Image Out"=w437:T1)  [unwired: 7 in]
        n217 = call "IMAQ Merge Overlay"("error in (no error)"=w438, "Image Src"=w437) -> ("Image Dst Out"=w433:T1)  [unwired: 8 in, 1 out]
      }
      frame "Forward" {
        n218 = call "IMAQ Overlay Bitmap"("Bitmap"=w439, "Top Left Point"=cluster{"X":i32, "Y":i32} {"X"=277, "Y"=423}, "Image"=w441) -> ("error out"=w444:errorcluster, "Image Out"=w443:T1)  [unwired: 7 in]
        n219 = call "IMAQ Merge Overlay"("error in (no error)"=w444, "Image Src"=w443) -> ("Image Dst Out"=w440:T1)  [unwired: 8 in, 1 out]
      }
    }
    "Image 2" <- w351
  }
